vi "Read Owner ID.vi"(11 "Properties in":refnum<class "Properties.lvclass">) -> (2 "owner-id":string, 3 "Properties out":refnum<class "Properties.lvclass">)   [LabVIEW 2013, in "Caraya.lvlib" / "Properties.lvclass"]
uses:
  Properties.lvclass
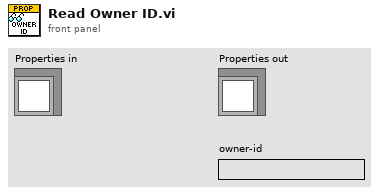
[diagram p1: front panel]
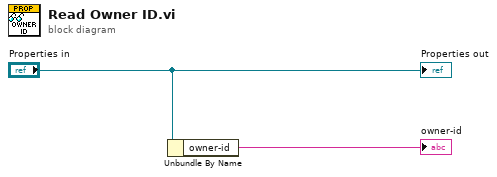
[diagram p0: block diagram]
diagram:
  n1 = Unbundle By Name("Properties in") -> ("owner-id"=→"owner-id":string)
  "Properties out" <- "Properties in"
